vi "readrems.vi"() -> ()   [LabVIEW 2010]
uses:
  <vilib>/Utility/config.llb/NI_LVConfig.lvlib
  <vilib>/addons/internet/NI_InternetTK_Core_VIs.lvlib
panel:
  out "message":string
  in  "SrcURL":string
  in  "DevNo":i32=10
  out "Rezult":string
  out "date/time":string
  in  "RunTwice":bool=TRUE
  in  "CMDpath":path
  in  "ReplyTo":string
  in  "WDTpath":path
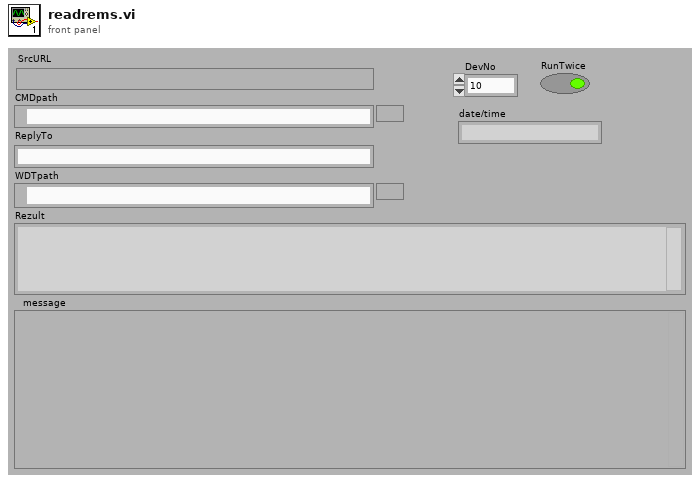
[diagram p1: front panel]
types:
  T1 = typedef "NI_LVConfig.lvlib/Config Data RefNum.ctl" = refnum<k1>
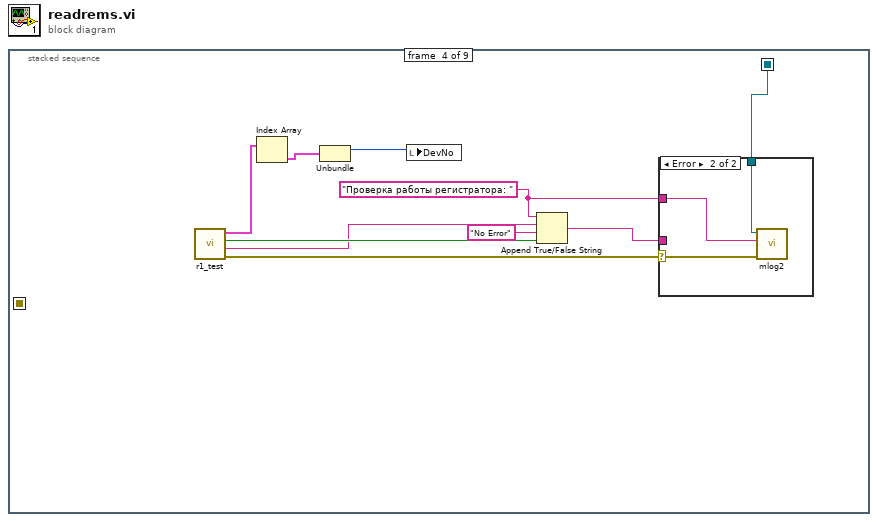
[diagram p0: block diagram]
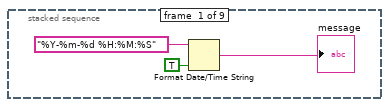
[diagram p2: hidden frame]
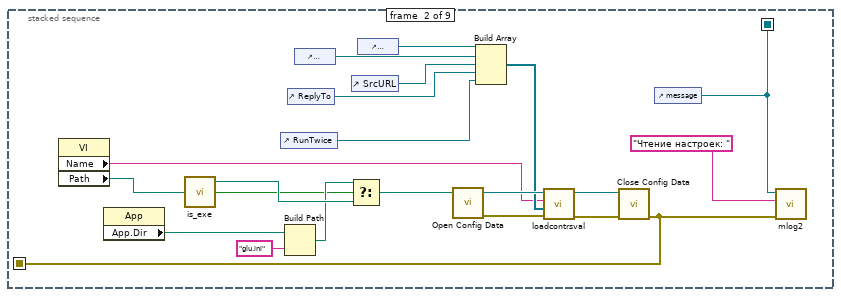
[diagram p3: hidden frame]
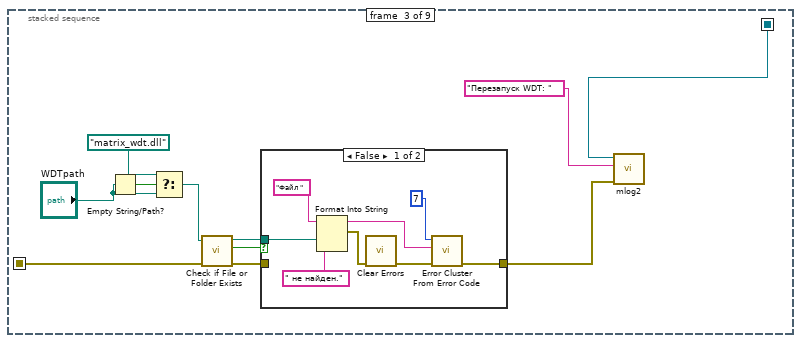
[diagram p4: hidden frame]
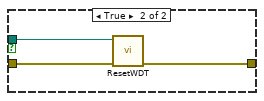
[diagram p5: hidden frame]
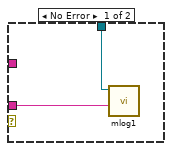
[diagram p6: hidden frame]
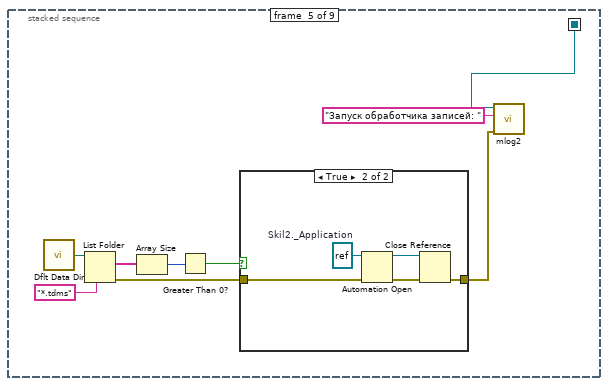
[diagram p7: hidden frame]
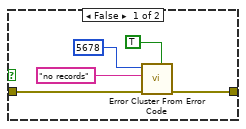
[diagram p8: hidden frame]
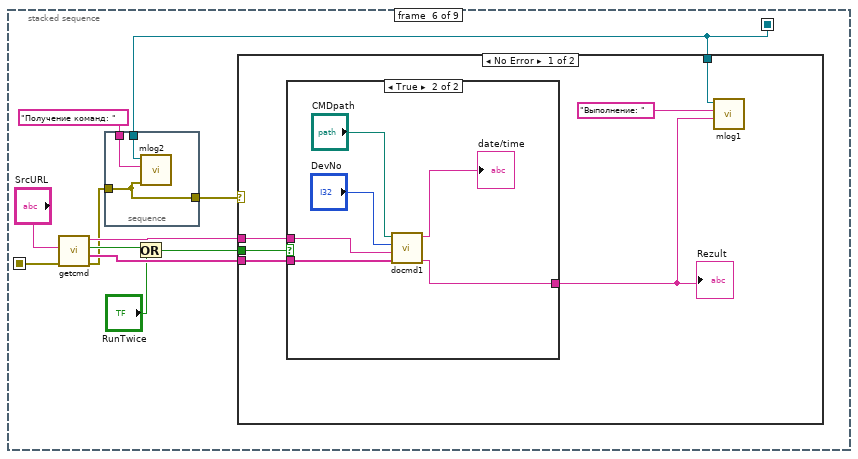
[diagram p9: hidden frame]
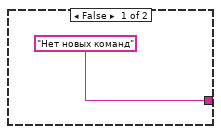
[diagram p10: hidden frame]
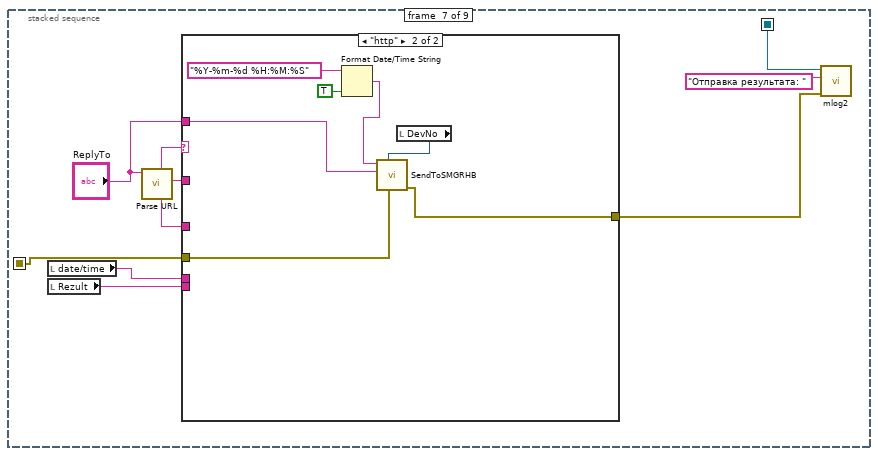
[diagram p12: hidden frame]
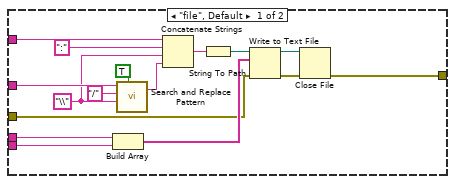
[diagram p13: hidden frame]
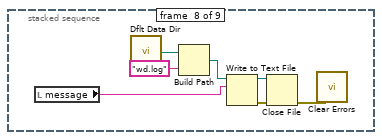
[diagram p14: hidden frame]
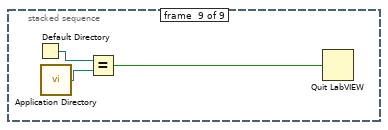
[diagram p15: hidden frame]
diagram:
  n1 = stacked-sequence {
    seq-local: [_ w4 _ _ _ _ _ _ _] -> [_ _ w32 _ _ w90 w108 _ _]
    seq-local: [_ w6 _ _ _ _ _ _ _] -> [_ _ w34 w53 w64 w82 w112 _ _]
    frame #0 {
      n2 = Format Date/Time String(time format string (%c)="%Y-%m-%d %H:%M:%S", UTC format=TRUE) -> (date/time string=→"message":string)  [unwired: 1 in]
    }
    frame #1 {
      n3 = property class="VI"() -> ("Name"=w17:string, "Path"=w14:path)  [unwired: 2 in, 2 out]
      n4 = property class="App"() -> ("App.Dir"=w10:path)  [unwired: 2 in, 2 out]
      n5 = call "is_exe.vi"("path"=w14) -> ("exe?"=w7:bool, "ini path"=w13:path)  [unwired: 2 in, 1 out]
      n6 = control-ref of="RunTwice"() -> (w9:refnum<vi>)
      n7 = Build Path(base path=w10, name or relative path="glu.ini") -> (appended path=w12:path)
      n8 = control-ref of="ReplyTo"() -> (w15:refnum<vi>)
      n9 = control-ref of="CMDpath"() -> (w22:refnum<vi>)
      n10 = Select(t=w12, s=w7, f=w13) -> (s? t:f=w11:path)
      n11 = control-ref of="SrcURL"() -> (w16:refnum<vi>)
      n12 = control-ref of="WDTpath"() -> (w8:refnum<vi>)
      n13 = call <vilib>:"Open Config Data.vi"("configuration file path"=w11) -> ("error out"=w24:errorcluster, "refnum"=w23:T1)  [unwired: 8 in, 1 out]
      n14 = Build Array(w8, w22, w16, w15, w9) -> (w21:refnum<vi>[])
      n15 = call "loadcontrsval.vi"("error in"=w24, "Array"=w21, "Section"=w17, "refnum in"=w23) -> ("error out"=w19:errorcluster, "refnum out"=w20:T1)  [unwired: 1 in, 1 out]
      n16 = call <vilib>:"Close Config Data.vi"("error in (no error)"=w19, "refnum"=w20) -> ("error out"=w4:errorcluster)  [unwired: 8 in, 1 out]
      n17 = control-ref of="message"() -> (w6:refnum<vi>)
      n18 = call "mlog2.vi"("reference"=w6, "String"="Чтение настроек: ", "error in"=w4) -> ()  [unwired: 5 in]
    }
    frame #2 {
      n19 = Empty String/Path?(string/path="WDTpath") -> (empty?=w28:bool)
      n20 = Select(t=path "matrix_wdt.dll" ("WDTpath"), s=w28, f="WDTpath") -> (s? t:f=w26:path)
      n21 = call <vilib>:"Check if File or Folder Exists.vi"("error in (no error)"=w32, "path"=w26) -> ("error out"=w30:errorcluster, "file or folder exists?"=w31:bool, "dup path"=w29:path)  [unwired: 7 in]
      n22 = case shown="False" w31 {
        tunnel: [w43 w46] -> w35
        tunnel: w30 -> [_ w45]
        tunnel: w29 -> [w41 w44]
        frame False {
          n23 = Format Into String(initial string="Файл ", w41, " не найден.") -> (resulting string=w38:string, error out=w37:errorcluster)  [unwired: 2 in]
          n24 = call <vilib>:"Clear Errors.vi"("error in (no error)"=w37) -> ("error out"=w36:errorcluster)  [unwired: 6 in]
          n25 = call <vilib>:"Error Cluster From Error Code.vi"("error in (no error)"=w36, "error message (\"\")"=w38, "error code (0)"=7) -> ("error out"=w43:errorcluster)  [unwired: 6 in]
        }
        frame True {
          n26 = call "ResetWDT.vi"("error in (no error)"=w45, "path in"=w44) -> ("error out"=w46:errorcluster)  [unwired: 4 in, 1 out]
        }
      }
      n27 = call "mlog2.vi"("reference"=w34, "String"="Перезапуск WDT: ", "error in"=w35) -> ()  [unwired: 5 in]
    }
    frame #3 {
      w47 = "Проверка работы регистратора: "
      n28 = call "r1_test.vi"() -> ("error out"=w52:errorcluster, "reason"=w49:string, "errr"=w50:bool, "devs"=w56:cluster{i32, string}[])  [unwired: 4 in]
      n29 = Index Array(array=w56) -> (element=w55:cluster{i32, string})  [unwired: 1 in]
      n30 = Unbundle(w55) -> (w54:i32)  [unwired: 1 out]
      n31 = local write "DevNo"(w54) -> ()
      n32 = Append True/False String(1:w50, 2:"No Error" ("false string"), 3:w49, 4:w47) -> (0:w51:string)
      n33 = case shown="Error" w52 {
        selector: w52 -> [_ w60]
        tunnel: w51 -> [w57 _]
        tunnel: w53 -> [w58 w61]
        tunnel: w47 -> [_ w59]
        frame No Error {
          n34 = call "mlog1.vi"("string2"=w57, "message"=w58) -> ()  [unwired: 6 in]
        }
        frame Error {
          n35 = call "mlog2.vi"("reference"=w61, "String"=w59, "error in"=w60) -> ()  [unwired: 5 in]
        }
      }
    }
    frame #4 {
      n36 = call <vilib>:"Dflt Data Dir.vi"() -> ("App:Default Data Directory"=w70:path)
      n37 = List Folder(path=w70, pattern="*.tdms") -> (filenames=w68:string[], error out=w65:errorcluster)  [unwired: 2 in, 2 out]
      n38 = Array Size(array=w68) -> (size(s)=w67:i32)
      n39 = Greater Than 0?(x=w67) -> (x > 0?=w62:bool)
      n40 = case shown="True" w62 {
        tunnel: [w75 w77] -> w66
        tunnel: w65 -> [w71 w76]
        frame False {
          n41 = call <vilib>:"Error Cluster From Error Code.vi"("is warning? (False)"=TRUE, "error in (no error)"=w71, "error message (\"\")"="no records" ("error message (\"\")"), "error code (0)"=5678) -> ("error out"=w75:errorcluster)  [unwired: 5 in]
        }
        frame True {
          w78 = refnum<k7> refnum  # Skil2._Application
          n42 = Automation Open(error in (no error)=w76, Automation Refnum=w78) -> (Automation Refnum=w79:refnum<k7>, error out=w80:errorcluster)  [unwired: 2 in]
          n43 = Close Reference(reference=w79, error in (no error)=w80) -> (error out=w77:errorcluster)
        }
      }
      n44 = call "mlog2.vi"("reference"=w64, "String"="Запуск обработчика записей: ", "error in"=w66) -> ()  [unwired: 5 in]
    }
    frame #5 {
      n45 = call "getcmd.vi"("error in"=w90, "srcurl"="SrcURL") -> ("error out"=w84:errorcluster, "Elements"=w91:string[], "new?"=w86:bool, "lowercase file ext"=w89:string)  [unwired: 2 in]
      n46 = stacked-sequence {
        tunnel: w84 -> [w92]
        tunnel: "Получение команд: " ("String") -> [w94]
        tunnel: w82 -> [w93]
        tunnel: [w92] -> w81
        frame #0 {
          n47 = call "mlog2.vi"("reference"=w93, "String"=w94, "error in"=w92) -> ()  [unwired: 5 in]
        }
      }
      n48 = Or(x=w86, y="RunTwice") -> (x .or. y?=w85:bool)
      n49 = case shown="No Error" w81 {
        tunnel: w91 -> [w100 _]
        tunnel: w89 -> [w99 _]
        tunnel: w85 -> [w98 _]
        tunnel: w82 -> [w97 _]
        frame No Error {
          n50 = case shown="True" w98 {
            tunnel: w100 -> [_ w107]
            tunnel: w99 -> [_ w106]
            tunnel: ["Нет новых команд" ("error message (\"\")") w102] -> w95
            frame False {
            }
            frame True {
              n51 = call "docmd1.vi"("Elements"=w107, "lowercase file ext"=w106, "DevNo"="DevNo", "CMDpath"="CMDpath") -> ("rezult"=w102:string, "date_time"=→"date/time":string)  [unwired: 1 in, 1 out]
            }
          }
          "Rezult" <- w95
          n52 = call "mlog1.vi"("string2"=w95, "string1"="Выполнение: ", "message"=w97) -> ()  [unwired: 5 in]
        }
        frame Error {
        }
      }
    }
    frame #6 {
      n53 = local read "date/time"() -> (w110:string)
      n54 = local read "Rezult"() -> (w109:string)
      n55 = call <vilib>:"Parse URL.vi"("URL"="ReplyTo") -> ("host"=w116:string, "virtual path"=w114:string, "protocol"=w117:string)  [unwired: 5 in, 3 out]
      n56 = case shown="\"http\"" w117 {
        tunnel: w116 -> [w127 _]
        tunnel: "ReplyTo" -> [_ w140]
        tunnel: w114 -> [w128 _]
        tunnel: [w122 w138] -> w113
        tunnel: w110 -> [w121 _]
        tunnel: w109 -> [w119 _]
        tunnel: w108 -> [w118 w139]
        frame "file", Default {
          w123 = "\\" ("replace string (\"\")")
          n57 = Build Array(w121, w119) -> (w120:string[])
          n58 = call <vilib>:"Search and Replace Pattern.vi"("string"=w128, "regular expression (\"\")"="/" ("regular expression (\"\")"), "replace string (\"\")"=w123, "replace all? (F)"=TRUE) -> ("result string"=w124:string)  [unwired: 1 in, 1 out]
          n59 = Concatenate Strings(w127, ":" ("string"), w123, w124) -> (w126:string)
          n60 = String To Path(string=w126) -> (path=w129:path)
          n61 = Write to Text File(file (use dialog)=w129, text=w120, error in=w118) -> (refnum out=w130:refnum<file>, error out=w131:errorcluster)  [unwired: 1 in, 1 out]
          n62 = Close File(refnum=w130, error in=w131) -> (error out=w122:errorcluster)  [unwired: 1 out]
        }
        frame "http" {
          n63 = Format Date/Time String(time format string (%c)="%Y-%m-%d %H:%M:%S", UTC format=TRUE) -> (date/time string=w134:string)  [unwired: 1 in]
          n64 = local read "DevNo"() -> (w137:i32)
          n65 = call "SendToSMGRHB.vi"("error in"=w139, "meas_point"=w137, "URL"=w140, "date"=w134) -> ("error out"=w138:errorcluster)  [unwired: 5 in, 2 out]
        }
      }
      n66 = call "mlog2.vi"("reference"=w112, "String"="Отправка результата: ", "error in"=w113) -> ()  [unwired: 5 in]
    }
    frame #7 {
      n67 = local read "message"() -> (w142:string)
      n68 = call <vilib>:"Dflt Data Dir.vi"() -> ("App:Default Data Directory"=w145:path)
      n69 = Build Path(base path=w145, name or relative path="wd.log") -> (appended path=w144:path)
      n70 = Write to Text File(file (use dialog)=w144, text=w142) -> (refnum out=w147:refnum<file>, error out=w143:errorcluster)  [unwired: 2 in, 1 out]
      n71 = Close File(refnum=w147, error in=w143) -> (error out=w141:errorcluster)  [unwired: 1 out]
      n72 = call <vilib>:"Clear Errors.vi"("error in (no error)"=w141) -> ()  [unwired: 6 in, 1 out]
    }
    frame #8 {
      n73 = Default Directory() -> (w149:path)
      n74 = call <vilib>:"Application Directory.vi"() -> ("Application Directory"=w150:path)
      n75 = Equal?(x=w149, y=w150) -> (x = y?=w148:bool)
      n76 = Quit LabVIEW(quit? (T)=w148) -> ()
    }
  }
